vi "filter.test.vi"(9 "reset":bool, 10 "debug":bool) -> ()   [LabVIEW 2020]
uses:
  <vilib>/Platform/TimedLoop/XDataNode/timing_clust.ctl
  <vilib>/Platform/TimedLoop/XDataNode/nitl_modes.ctl
  <vilib>/Platform/TimedLoop/XDataNode/wakeup.ctl
  ticker.slot.ctl
  common/orderbook.command.ctl
  common/orderbook.command.type.ctl
  <vilib>/rvi/Emulation/niFpgaSctlEmulationGetInTimedLoop.vi
  <vilib>/rvi/Emulation/niFpgaEmulationReportErrorSimple.vi
  <vilib>/rvi/Emulation/niFpgaGetClockAttributes.vi
  <vilib>/rvi/Emulation/niFpgaCriticalErrorInLSC.vi
  <vilib>/rvi/Emulation/niFpgaEmulationIsFPGAContextNoSignature.vi
  <vilib>/rvi/errors/niFpgaSetErrorForExecOnDevCompSimple.vi
  <vilib>/rvi/eio/common/nirviEmuReportErrorAndStop.vi
  <vilib>/rvi/DataTransferAndStorage/Container/Common/niFpgaContainerGetUniqueNameForEmu.vi
  <vilib>/rvi/FIFO/Fifo_Resource/nirvififoEmulationSetSize.vi
  <vilib>/rvi/FIFO/Fifo_Resource/nirviFifoEmulationQueueMgr.vi
  <instcachedir>/0/nirviFifoEmulationQueueMgr_E5CAEC123FF24DC58D834DCA3CDAA9B5.lvgen/nirviFifoEmulationQueueMgr_E5CAEC123FF24DC58D834DCA3CDAA9B5_008.vi
  <vilib>/Utility/error.llb/Clear Errors.vi
  <vilib>/rvi/FIFO/Fifo_Resource/nirvififoEmulationCreateLock.vi
  <vilib>/rvi/Emulation/niFpgaProcessEmulError.vi
  <vilib>/rvi/FIFO/Fifo_Resource/nirvififoEmulationObtainLock.vi
  <vilib>/rvi/FIFO/Fifo_Resource/nirvififoEmulationReleaseLock.vi
  <vilib>/rvi/occurrence/nirviWaitOnOccurrenceBase.vi
  <vilib>/rvi/errors/nirviReportUnexpectedCaseInternalError.vi
  <vilib>/rvi/errors/nirviReportUnexpectedCaseInternalError (U32).vi
  <vilib>/rvi/interface/RandomDataEmulation/nirviRandomDataMultiElementFPGAFIFO.vi
  <instcachedir>/0/nirviRandomDataMultiElementFPGAFIFO_3E9965BA1FAD4E7B8DABA31768A09B1F.lvgen/nirviRandomDataMultiElementFPGAFIFO_3E9965BA1FAD4E7B8DABA31768A09B1F_001.vi
  <vilib>/rvi/interface/RandomDataEmulation/niFpgaRandomDataHandleErrors.vi
  <instcachedir>/0/nirviFifoEmulationQueueMgr_E5CAEC123FF24DC58D834DCA3CDAA9B5.lvgen/nirviFifoEmulationQueueMgr_E5CAEC123FF24DC58D834DCA3CDAA9B5_007.vi
  <vilib>/rvi/FIFO/Fifo_Resource/nirvififoEmulationDetermineInputValidOut.vi
  <vilib>/rvi/DataTransferAndStorage/Container/Common/niFpgaContainerSetEmuInfo.vi
  <vilib>/rvi/DataTransferAndStorage/Container/Common/niFpgaContainerExecOnDevCompGetState.vi
  <instcachedir>/0/nirviFifoEmulationQueueMgr_E5CAEC123FF24DC58D834DCA3CDAA9B5.lvgen/nirviFifoEmulationQueueMgr_E5CAEC123FF24DC58D834DCA3CDAA9B5_009.vi
  <vilib>/Platform/TimedLoop/XDataNode/XDataNode.xnode
  <vilib>/rvi/DataTransferAndStorage/Container/XNode/niFpgaContainer.xnode
  <vilib>/rvi/FIFO/Fifo_Resource/nirvififoEmulationRead.vi
  <vilib>/rvi/interface/RandomDataEmulation/nirviRandomDataFpgaMultiElementTemplate.vi
  <vilib>/rvi/FIFO/Fifo_Resource/nirvififoEmulationWrite.vi
  <vilib>/rvi/LocalResourceManager/LocalResourceManager.xnode
  <vilib>/rvi/FIFO/Fifo_Resource/niFpgaFifoEmulationRefIn.vi
  <vilib>/rvi/interface/RandomDataEmulation/nirviRandomDataFpgaReadWriteTemplate.vi
  <vilib>/Platform/TimedLoop/XDataNode/XDNodeRunTimeDep.lvlib
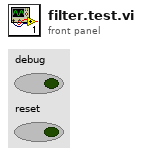
[diagram p1: front panel]
types:
  T1 = typedef "XDNodeRunTimeDep.lvlib/timing_clust.ctl" = cluster{"Expected End [f-1]":u64, "Actual End [f-1]":u64, "Finished Late? [f-1]":bool, "Expected End [i-1]":u64, "Actual End [i-1]":u64, "Finished Late? [i-1]":bool, "Expected Start [i]":u64, "Actual Start [i]":u64, "Expected Start [f]":u64, "Actual Start [f]":u64, "Source Name":string, "Structure Name":string, "Period":i64, "Deadline":i64, "Offset":i64, "Start":i64, "Priority":i32, "Timeout":i32, "Mode":T2, "Wakeup Reason":T3, "Error":errorcluster, "Source Type":string, "Secondary Source Type":string, "Global End Time":u64, "Global Start Time":u64, "Frame Duration":u64, "Iteration Duration":u64, "Assigned CPU":i32, "I/O Scan Engine Mode":u32}
  T2 = typedef "XDNodeRunTimeDep.lvlib/nitl_modes.ctl" = enum32{"No Change", "Process missed periods, maintain original phase", "Discard missed periods, maintain original phase", "Process missed periods, ignore original phase", "Discard missed periods, ignore original phase"}
  T3 = typedef "XDNodeRunTimeDep.lvlib/wakeup.ctl" = enum32{"Normal", "Aborted", "Asynchronous wakeup", "Timing source error", "Timed loop error", "Timeout"}
  T4 = typedef "orderbook.command.ctl" = cluster{"type":T5, "side":u8, "orderId ":u64, "quantity":u32, "symbol":u64, "price":u64, "executed.qty":u32, "canceled.qty":u32, "remaining.qty":u32, "seconds":u64, "nanoseconds":u64, "Add":bool, "Edit":bool, "Remove":bool}
  T5 = typedef "orderbook.command.type.ctl" = enum8{"Time", "AddOrder", "OrderExecuted", "OrderExecutedAtPrice", "ReduceSize", "ModifyOrder", "DeleteOrder", "Get.Everything", "Get.All.Orders", "Get.Top"}
  T6 = typedef "ticker.slot.ctl" = cluster{"Symbol":u64}
  T7 = cluster{"type":enum8{"Time", "AddOrder", "OrderExecuted", "OrderExecutedAtPrice", "ReduceSize", "ModifyOrder", "DeleteOrder", "Get.Everything", "Get.All.Orders", "Get.Top"}, "side":u8, "orderId ":u64, "quantity":u32, "symbol":u64, "price":u64, "executed.qty":u32, "canceled.qty":u32, "remaining.qty":u32, "seconds":u64, "nanoseconds":u64, "Add":bool, "Edit":bool, "Remove":bool}
  T8 = enum8{"Time", "AddOrder", "OrderExecuted", "OrderExecutedAtPrice", "ReduceSize", "ModifyOrder", "DeleteOrder", "Get.Everything", "Get.All.Orders", "Get.Top"}
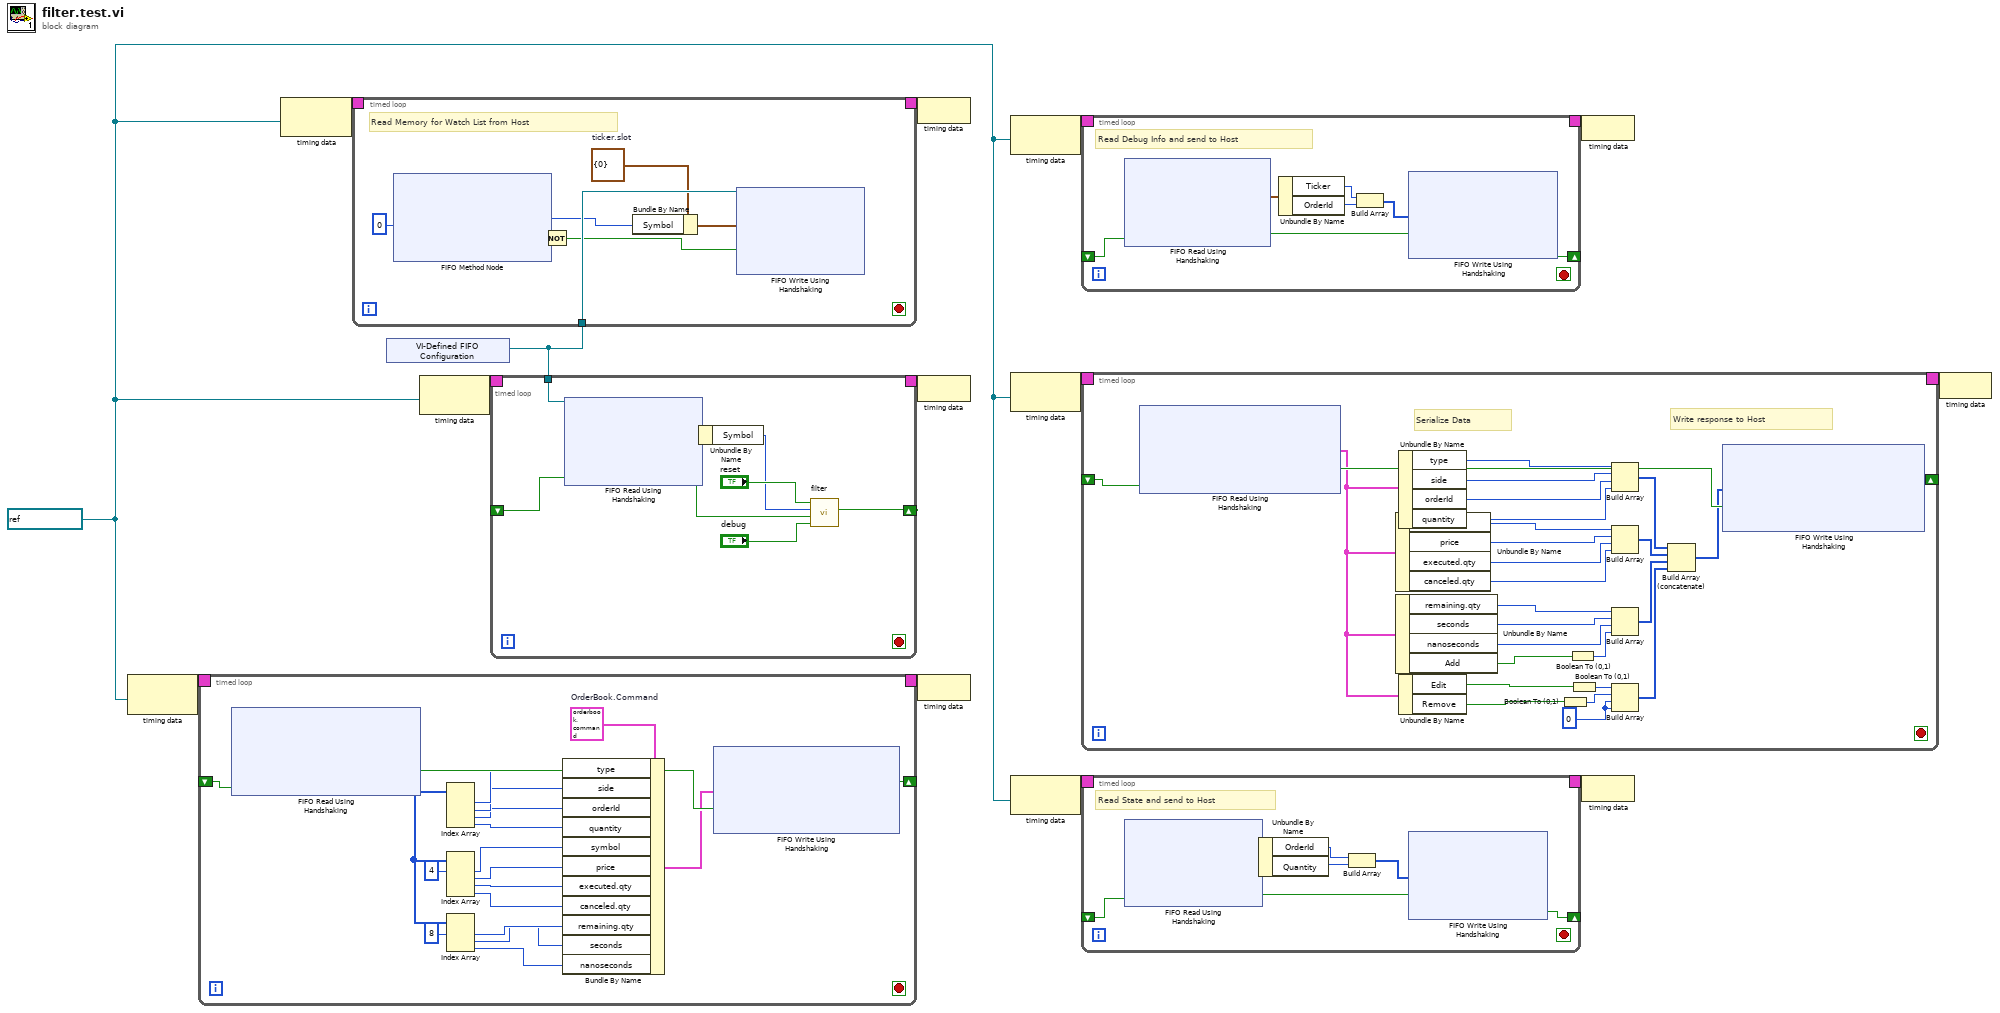
[diagram p0: block diagram]
diagram:
  w1 = refnum<k21> "160MHz" ("Source Name")
  n1 = node-c288(w1) -> (w7:T1)
  n2 = timed-loop {
    timing: w7 -> [_]
    timing-out: [_] -> w6
    shift-right: [w33] -> _
    shift-left: _ -> [w32]
    stop <- _ stop-if-true
    w30 = T4 {"type"=enum."AddOrder", "side"=0, "orderId "=0, "quantity"=0, "symbol"=0, "price"=0, "executed.qty"=0, "canceled.qty"=0, "remaining.qty"=0, "seconds"=0, "nanoseconds"=0, "Add"=FALSE, "Edit"=FALSE, "Remove"=FALSE}  # OrderBook.Command
    n3 = xnode ("FIFO Read Using Handshaking")("Ready for Output"=w32) -> ("Element"=w28:u64[], "Output Valid"=w31:bool)  [unwired: 1 in, 1 out]
    n4 = Index Array(array=w28) -> (element #1=w25:u64, element #2=w24:u64, element #3=w23:u64, element #4=w22:u64)  [unwired: 4 in]
    n5 = Index Array(array=w28, index #1=4 ("index")) -> (element #1=w21:u64, element #2=w20:u64, element #3=w19:u64, element #4=w18:u64)  [unwired: 3 in]
    n6 = Index Array(array=w28, index #1=8 ("index")) -> (element #1=w17:u64, element #2=w16:u64, element #3=w15:u64)  [unwired: 2 in]
    n7 = Bundle By Name(cluster=w30, "type"=w25, "side"=w24, "orderId"=w23, "quantity"=w22, "symbol"=w21, "price"=w20, "executed.qty"=w19, "canceled.qty"=w18, "remaining.qty"=w17, "seconds"=w16, "nanoseconds"=w15) -> (w29:T4)
    n8 = xnode ("FIFO Write Using Handshaking")("Element"=w29, "Input Valid"=w31) -> ("Ready for Input"=w33:bool)  [unwired: 1 in, 1 out]
  }
  n9 = node-c288(w1) -> (w12:T1)
  n10 = xnode "VI-Defined FIFO Configuration"() -> ("FIFO Out"=w10:refnum<k21>)
  n11 = timed-loop {
    timing: w12 -> [_]
    timing-out: [_] -> w11
    tunnel: w10 -> [w41]
    stop <- _ stop-if-true
    w38 = T6 {"Symbol"=0}  # ticker.slot
    # "Read Memory for Watch List from Host"
    n12 = xnode ("FIFO Method Node")("Timeout"=0) -> ("Element"=w36:u64, "Timed Out?"=w40:bool)  [unwired: 1 in, 1 out]
    n13 = Not(x=w40) -> (.not. x?=w39:bool)
    n14 = Bundle By Name(cluster=w38, "Symbol"=w36) -> (w37:T6)
    n15 = xnode ("FIFO Write Using Handshaking")("Element"=w37, "Input Valid"=w39, "FIFO In"=w41) -> ()  [unwired: 2 out]
  }
  n16 = node-c288(w1) -> (w14:T1)
  n17 = timed-loop {
    timing: w14 -> [_]
    timing-out: [_] -> w13
    tunnel: w10 -> [w52]
    shift-right: [w47] -> _
    shift-left: _ -> [w46]
    stop <- _ stop-if-true
    n18 = xnode ("FIFO Read Using Handshaking")("Ready for Output"=w46, "FIFO In"=w52) -> ("Element"=w51:cluster{"Symbol":u64}, "Output Valid"=w49:bool)  [unwired: 1 out]
    n19 = Unbundle By Name(w51) -> ("Symbol"=w45:u64)
    n20 = call "filter.vi"("debug"="debug", "conf.valid"=w49, "conf"=w45, "reset"="reset") -> ("Ready.for.Configuration.Input"=w47:bool)  [unwired: 6 in, 1 out]
  }
  n21 = node-c288(w11) -> ()
  n22 = node-c288(w13) -> ()
  n23 = node-c288(w6) -> ()
  n24 = node-c288(w1) -> (w9:T1)
  n25 = node-c288(w1) -> (w5:T1)
  n26 = node-c288(w1) -> (w3:T1)
  n27 = timed-loop {
    timing: w9 -> [_]
    timing-out: [_] -> w8
    shift-right: [w61] -> _
    shift-left: _ -> [w60]
    stop <- _ stop-if-true
    # "Read Debug Info and send to Host"
    n28 = xnode ("FIFO Read Using Handshaking")("Ready for Output"=w60) -> ("Element"=w58:cluster{"Ticker":u64, "OrderId":u64}, "Output Valid"=w59:bool)  [unwired: 1 in, 1 out]
    n29 = Unbundle By Name(w58) -> ("Ticker"=w56:u64, "OrderId"=w57:u64)
    n30 = Build Array(w56, w57) -> (w55:u64[])
    n31 = xnode ("FIFO Write Using Handshaking")("Element"=w55, "Input Valid"=w59) -> ("Ready for Input"=w61:bool)  [unwired: 1 in, 1 out]
  }
  n32 = timed-loop {
    timing: w5 -> [_]
    timing-out: [_] -> w4
    shift-right: [w90] -> _
    shift-left: _ -> [w85]
    stop <- _ stop-if-true
    w67 = u64 0 ("element")
    # "Serialize Data"
    # "Write response to Host"
    n33 = xnode ("FIFO Read Using Handshaking")("Ready for Output"=w85) -> ("Element"=w70:T7, "Output Valid"=w84:bool)  [unwired: 1 in, 1 out]
    n34 = Unbundle By Name(w70) -> ("symbol"=w89:u64, "price"=w88:u64, "executed.qty"=w87:u32, "canceled.qty"=w86:u32)
    n35 = Unbundle By Name(w70) -> ("remaining.qty"=w80:u32, "seconds"=w78:u64, "nanoseconds"=w79:u64, "Add"=w76:bool)
    n36 = Unbundle By Name(w70) -> ("type"=w68:T8, "side"=w66:u8, "orderId"=w65:u64, "quantity"=w64:u32)
    n37 = Unbundle By Name(w70) -> ("Edit"=w74:bool, "Remove"=w72:bool)
    n38 = Boolean To (0,1)(Boolean=w72) -> (0, 1=w71:i16)
    n39 = Boolean To (0,1)(Boolean=w76) -> (0, 1=w75:i16)
    n40 = Boolean To (0,1)(Boolean=w74) -> (0, 1=w73:i16)
    n41 = Build Array(w68, w66, w65, w64) -> (w69:u64[])
    n42 = Build Array(w89, w88, w87, w86) -> (w83:u64[])
    n43 = Build Array(w80, w78, w79, w75) -> (w81:u64[])
    n44 = Build Array(w73, w71, w67, w67) -> (w77:u64[])
    n45 = Build Array (concatenate)(w69, w83, w81, w77) -> (w82:u64[])
    n46 = xnode ("FIFO Write Using Handshaking")("Element"=w82, "Input Valid"=w84) -> ("Ready for Input"=w90:bool)  [unwired: 1 in, 1 out]
  }
  n47 = timed-loop {
    timing: w3 -> [_]
    timing-out: [_] -> w2
    shift-right: [w99] -> _
    shift-left: _ -> [w98]
    stop <- _ stop-if-true
    # "Read State and send to Host"
    n48 = xnode ("FIFO Read Using Handshaking")("Ready for Output"=w98) -> ("Element"=w96:cluster{"OrderId":u64, "Quantity":u64}, "Output Valid"=w97:bool)  [unwired: 1 in, 1 out]
    n49 = Unbundle By Name(w96) -> ("OrderId"=w95:u64, "Quantity"=w93:u64)
    n50 = Build Array(w95, w93) -> (w94:u64[])
    n51 = xnode ("FIFO Write Using Handshaking")("Element"=w94, "Input Valid"=w97) -> ("Ready for Input"=w99:bool)  [unwired: 1 in, 1 out]
  }
  n52 = node-c288(w8) -> ()
  n53 = node-c288(w2) -> ()
  n54 = node-c288(w4) -> ()
